vi "Get_SLOPE_data_from_file 2016.vi"(0 "Slopes File Path":path=path "C:/Cascade/Data/Output Files/slopes.csv") -> (3 "Last Aux 1 Slope":dbl, 4 "Output_array":sgl[][](array[numeric]) format="%.2f", 6 "Last_String_Pot_Slope":dbl format="%.2f", 7 "DHT Offset":dbl, 9 "DHT Slope":dbl, 10 "Last_Flow_Slope":dbl format="%.2f", 12 "Last Aux 2 Slope":dbl, 13 "APS tip distance to DHT":dbl, 14 "Last Aux 3 Slope":dbl, 15 "Last_Pressure_Slope":dbl format="%.2f")   [LabVIEW 2016]
uses:
  <vilib>/Utility/file.llb/Read Delimited Spreadsheet (DBL).vi
  <vilib>/Utility/file.llb/Read Delimited Spreadsheet (string).vi
panel:
  out "last row":dbl[](array[numeric])
  out "In Range?":bool
  out "min columns":i32
  out "Slopes Out of Range":bool
  out "number of rows\n(including header)":i32
  out "first row":string[](array[string])
  out "file or folder exists?":bool
  out "error out":errorcluster
  out "Last_KPRO_Box_Number":dbl
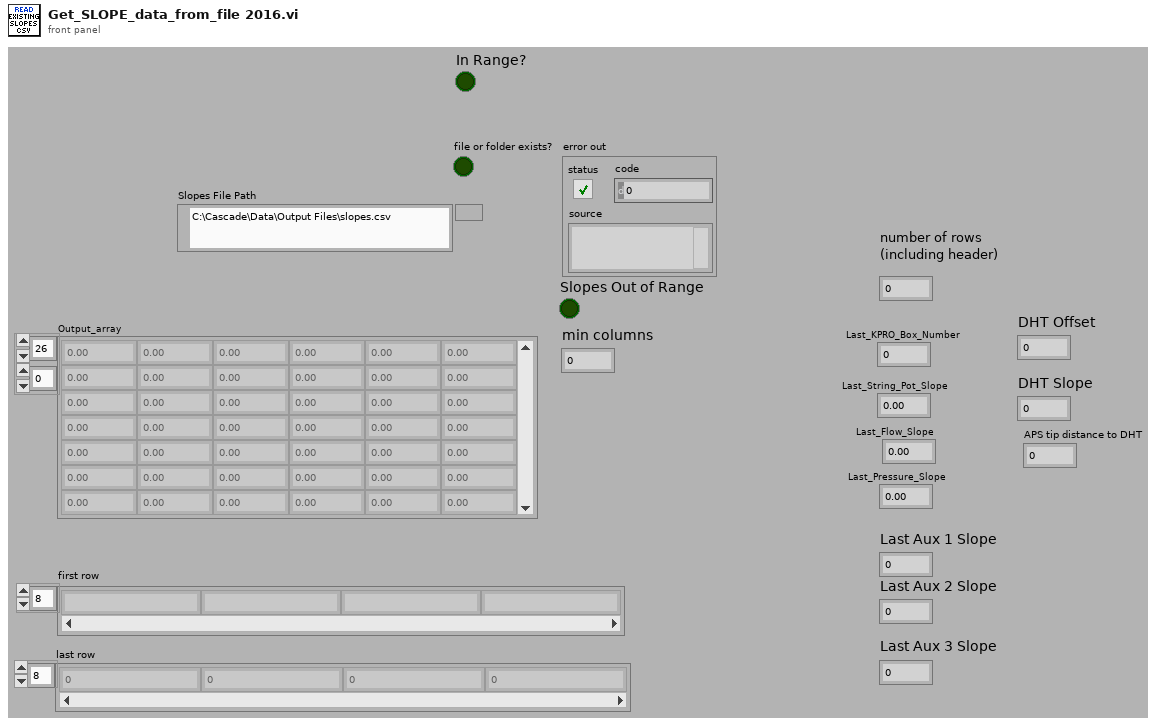
[diagram p1: front panel]
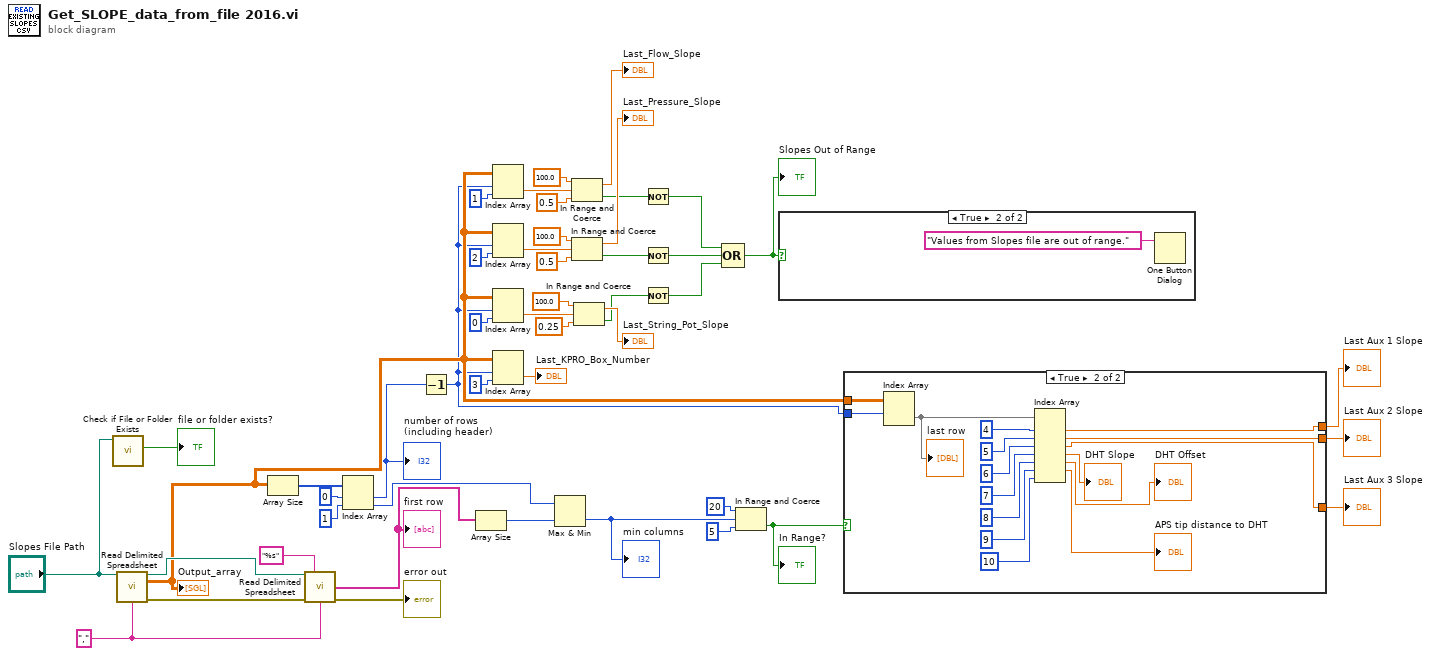
[diagram p0: block diagram]
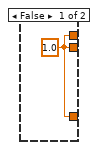
[diagram p3: hidden frame]
diagram:
  w41 = ","
  n1 = call <vilib>:"Check if File or Folder Exists.vi"("path"="Slopes File Path") -> ("file or folder exists?"=→"file or folder exists?":bool)  [unwired: 8 in, 2 out]
  n2 = call-poly <vilib>:"Read Delimited Spreadsheet.vi"("file path (dialog if empty)"="Slopes File Path", "delimiter (\\t)"=w41) -> ("new file path (Not A Path if cancelled)"=w45:path, "all rows"=w9:dbl[][], "error out"=w43:errorcluster)  [unwired: 8 in, 3 out]
  "Output_array" <- w9
  n3 = Array Size(array=w9) -> (size(s)=w36:i32[])
  n4 = call-poly <vilib>:"Read Delimited Spreadsheet.vi"("file path (dialog if empty)"=w45, "format (%s)"="%s" ("format (%.3f)"), "error in (no error)"=w43, "delimiter (\\t)"=w41) -> ("first row"=w40:string[], "error out"=→"error out":errorcluster)  [unwired: 6 in, 4 out]
  "first row" <- w40
  n5 = Index Array(array=w36, index #1=0 ("index"), index #2=1 ("index")) -> (element #1=w35:i32, element #2=w38:i32)
  "number of rows\n(including header)" <- w35
  n6 = Decrement(x=w35) -> (x-1=w4:i32)
  n7 = Array Size(array=w40) -> (size(s)=w39:i32)
  n8 = Index Array(array=w9, index (row)=w4, index (col)=1 ("disabled index (col)")) -> (element=w30:dbl)
  n9 = Index Array(array=w9, index (row)=w4, index (col)=2 ("index")) -> (element=w31:dbl)
  n10 = Index Array(array=w9, index (row)=w4, index (col)=0 ("index")) -> (element=w23:dbl)
  n11 = Index Array(array=w9, index (row)=w4, index (col)=3 ("index")) -> (element=→"Last_KPRO_Box_Number":dbl)
  n12 = Max & Min(x=w38, y=w39) -> (min(x,y)=w8:i32)  [unwired: 1 out]
  "min columns" <- w8
  n13 = In Range and Coerce(upper limit=100.0, x=w30, lower limit=0.5) -> (coerced(x)=→"Last_Flow_Slope":dbl, In Range?=w17:bool)
  n14 = In Range and Coerce(upper limit=100.0, x=w31, lower limit=0.5) -> (coerced(x)=→"Last_Pressure_Slope":dbl, In Range?=w16:bool)
  n15 = In Range and Coerce(upper limit=100.0, x=w23, lower limit=0.25) -> (coerced(x)=→"Last_String_Pot_Slope":dbl, In Range?=w15:bool)
  n16 = Not(x=w17) -> (.not. x?=w14:bool)
  n17 = Not(x=w16) -> (.not. x?=w13:bool)
  n18 = Not(x=w15) -> (.not. x?=w12:bool)
  n19 = Compound Arithmetic op=OR(w14, w13, w12) -> (w11:bool)
  "Slopes Out of Range" <- w11
  n20 = In Range and Coerce(upper limit=20, x=w8, lower limit=5) -> (In Range?=w5:bool)  [unwired: 1 out]
  "In Range?" <- w5
  n21 = case shown="True" w11 {
    frame False {
    }
    frame True {
      n22 = One Button Dialog(message="Values from Slopes file are out of range.") -> ()  [unwired: 1 in, 1 out]
    }
  }
  n23 = case shown="True" w5 {
    tunnel: w9 -> [_ w65]
    tunnel: w4 -> [_ w51]
    tunnel: [w49 w64] -> w3
    tunnel: [w49 w63] -> w2
    tunnel: [w49 w62] -> w1
    frame False {
      w49 = 1.0 ("Numeric")
    }
    frame True {
      n24 = Index Array(array=w65, index (row)=w51) -> (element=w57:dbl[])  [unwired: 1 in]
      "last row" <- w57
      n25 = Index Array(array=w57, index #1=4 ("disabled index (col)"), index #2=5 ("disabled index (col)"), index #3=6 ("disabled index (col)"), index #4=7 ("index (col)"), index #5=8 ("index (row)"), index #6=9 ("disabled index (row)"), index #7=10 ("disabled index (row)")) -> (element #1=w64:dbl, element #2=w63:dbl, element #3=w62:dbl, element #4=→"DHT Slope":dbl, element #5=→"DHT Offset":dbl, element #6=→"APS tip distance to DHT":dbl)  [unwired: 1 out]
    }
  }
  "Last Aux 1 Slope" <- w3
  "Last Aux 2 Slope" <- w2
  "Last Aux 3 Slope" <- w1
